vi "Value to Description.vi"(8 "error in":errorcluster, 11 "value":variant) -> (0 "error out":errorcluster, 2 "description":string, 3 "value out":variant)   [LabVIEW 2020, in "Value.lvlib"]
uses:
  Value.lvlib
  Display Metadata.ctl
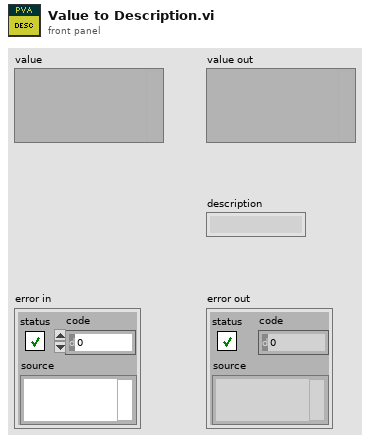
[diagram p1: front panel]
types:
  T1 = typedef "Value.lvlib/Display Metadata.ctl" = cluster{"Limit Low":dbl, "Limit High":dbl, "Description":string, "Units":string, "Precision":i32, "Form":enum32{"Default", "String", "Binary", "Decimal", "Hex", "Exponential", "Engineering"}}
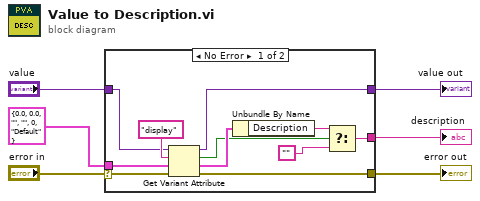
[diagram p0: block diagram]
diagram:
  n1 = case shown="No Error" "error in" {
    selector: "error in" -> [w15 w19]
    tunnel: [w12 w19] -> w6
    tunnel: "value" -> [w14 w18]
    tunnel: [w13 w18] -> w3
    tunnel: [w9 _] -> w2
    tunnel: T1 {"Limit Low"=0.0, "Limit High"=0.0, "Description"="", "Units"="", "Precision"=0, "Form"=enum."Default"} ("Display") -> [w8 _]
    frame No Error {
      n2 = Get Variant Attribute(Variant=w14, name="display", default value (empty Variant)=w8, error in=w15) -> (duplicate Variant=w13:variant, found=w11:bool, value=w17:T1, error out=w12:errorcluster)
      n3 = Unbundle By Name(w17) -> ("Description"=w10:string)
      n4 = Select(t=w10, s=w11, f="") -> (s? t:f=w9:string)
    }
    frame Error {
    }
  }
  "error out" <- w6
  "description" <- w2
  "value out" <- w3
